vi "Message lenght check.vi"(8 "error in (no error)":errorcluster, 10 "String in":string, 11 "TCP Writer in":refnum<class "TCP Writer.lvclass">) -> (0 "error out":errorcluster, 2 "String out":string, 3 "TCP Writer out":refnum<class "TCP Writer.lvclass">)   [LabVIEW 2026, in "TALOS.lvlib" / "TCP Writer.lvlib" / "TCP Writer.lvclass"]
uses:
  TCP Writer.lvclass
  Ancestor/Ancestor/Ancestor.lvclass/Ancestor.ctl
  FGV/Error Memory/Get Error Description.vi
  Support VIs/Get PC name.vi
  Ancestor/Ancestor/Read ID.vi
  Support VIs/Get Class Name.vi
  <vilib>/Utility/error.llb/Clear Errors.vi
  FGV/Error Memory/Error Memory Core.vi
  <vilib>/AdvancedString/Delimited String to 1D String Array.vi
  <vilib>/AdvancedString/Delimited String to 1D String Array (string).vi
  Support VIs/Circus Root Path.vi
  FGV/Error Memory/Error Crt Lvl checker.vi
  FGV/Error Memory/Error Memory Core.vi/40c8088d-b597-4017-91af-faa98e00292e.vi
  FGV/Error Memory/Error Memory Core.vi/d4a3ab98-063c-4e44-b43d-fbdcfe6c2be2.vi
  Support VIs/Global Constants.vi
  Support VIs/Global Memory.vi
  <vilib>/Utility/LVClass/Get LV Class Name.vi
  Support VIs/Is in Packed Library.vi
  Support VIs/TALOS Root path.vi
  Support VIs/Read CSV worksheet.vi
  <vilib>/Utility/error.llb/General Error Handler.vi
  Ancestor/Ancestor/Ancestor.lvclass
  <vilib>/Comparison/Equal/Equal Functor/Equal Functor.lvclass
  TALOS.lvlib
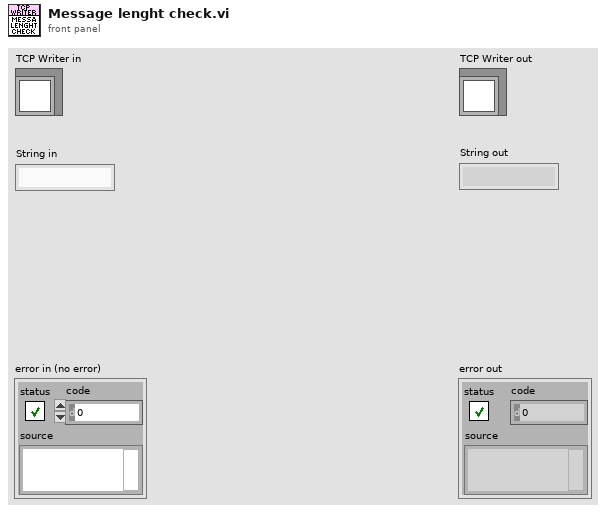
[diagram p1: front panel]
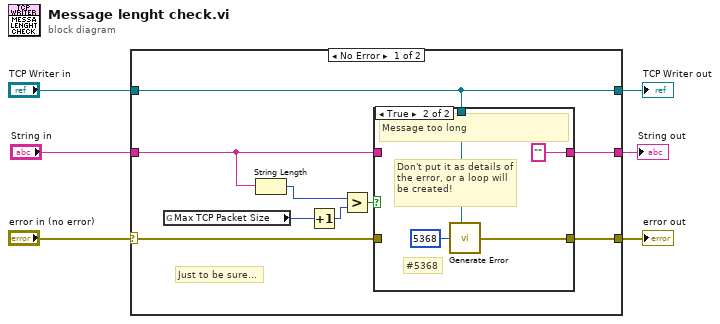
[diagram p0: block diagram]
diagram:
  n1 = case shown="No Error" "error in (no error)" {
    selector: "error in (no error)" -> [w14 w24]
    tunnel: [w11 w24] -> w5
    tunnel: [w10 w23] -> w3
    tunnel: "TCP Writer in" -> [w10 w23]
    tunnel: [w13 w22] -> w2
    tunnel: "String in" -> [w12 w22]
    frame No Error {
      # "Just to be sure..."
      n2 = global read "Global Constants.vi" "Max TCP Packet Size"() -> (w8:i32)
      n3 = String Length(string=w12) -> (length=w15:i32)
      n4 = Increment(x=w8) -> (x+1=w7:i32)
      n5 = Greater?(x=w15, y=w7) -> (0:w9:bool)
      n6 = case shown="True" w9 {
        tunnel: w14 -> [w16 _]
        tunnel: [w17 "" ("String in")] -> w13
        tunnel: w12 -> [w17 _]
        tunnel: [w16 w20] -> w11
        tunnel: w10 -> [_ w19]
        frame False {
          # "Length OK"
        }
        frame True {
          # "Don't put it as details of the error, or a loop will be created!"
          # "#5368"
          # "Message too long"
          n7 = call "Generate Error.vi"("Class"=w19, "Error Code"=5368) -> ("error out"=w20:errorcluster)  [unwired: 5 in]
        }
      }
    }
    frame Error {
    }
  }
  "error out" <- w5
  "TCP Writer out" <- w3
  "String out" <- w2
